vi "globalSetUp.vi"(8 "error in (no error)":errorcluster, 11 "testcase-CSMSyncMessage in":refnum<class "testcase-CSMSyncMessage.lvclass">) -> (0 "error out":errorcluster, 3 "testcase-CSMSyncMessage out":refnum<class "testcase-CSMSyncMessage.lvclass">)   [LabVIEW 2017, in "testcase-CSMSyncMessage.lvclass"]
uses:
  testcase-CSMSyncMessage.lvclass
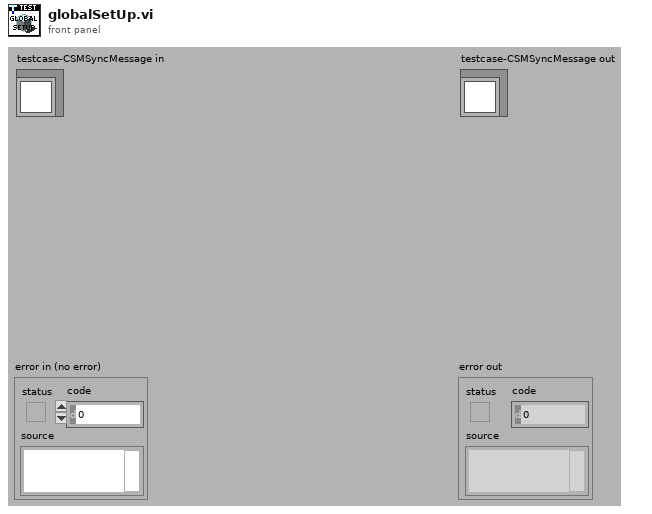
[diagram p1: front panel]
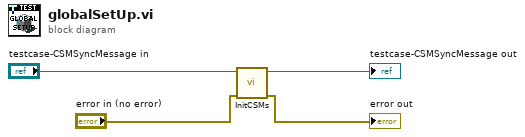
[diagram p0: block diagram]
diagram:
  n1 = call "InitCSMs.vi"("error in (no error)"="error in (no error)", "testcase-CSMSyncMessage in"="testcase-CSMSyncMessage in") -> ("error out"=→"error out":errorcluster, "testcase-CSMSyncMessage out"=→"testcase-CSMSyncMessage out":refnum<class "testcase-CSMSyncMessage.lvclass">)  [unwired: 8 in]
